vi "Beep.vi"(7 "Enable":bool=TRUE, 8 "Error In":errorcluster, 9 "Beep duration\n(sec)":dbl=0.15, 11 "Beep * n?":i32=1) -> (0 "Error Out":errorcluster)   [LabVIEW 2019]
uses:
  <vilib>/Platform/TimedLoop/XDataNode/timing_clust.ctl
  <vilib>/Platform/TimedLoop/XDataNode/nitl_modes.ctl
  <vilib>/Platform/TimedLoop/XDataNode/wakeup.ctl
  <vilib>/platform/TimedLoop/XDataNode/XDataNode.xnode
  WSCbot_V3_Toolkit.lvlibp
  <vilib>/Platform/TimedLoop/XDataNode/XDNodeRunTimeDep.lvlib
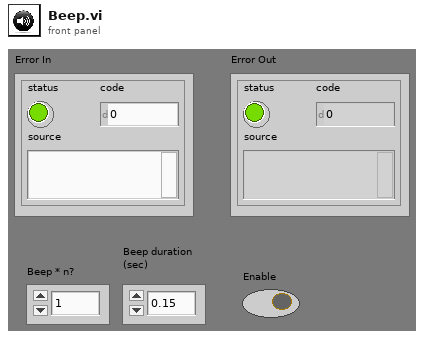
[diagram p1: front panel]
types:
  T1 = typedef "XDNodeRunTimeDep.lvlib/timing_clust.ctl" = cluster{"Expected End [f-1]":u64, "Actual End [f-1]":u64, "Finished Late? [f-1]":bool, "Expected End [i-1]":u64, "Actual End [i-1]":u64, "Finished Late? [i-1]":bool, "Expected Start [i]":u64, "Actual Start [i]":u64, "Expected Start [f]":u64, "Actual Start [f]":u64, "Source Name":string, "Structure Name":string, "Period":i64, "Deadline":i64, "Offset":i64, "Start":i64, "Priority":i32, "Timeout":i32, "Mode":T2, "Wakeup Reason":T3, "Error":errorcluster, "Source Type":string, "Secondary Source Type":string, "Global End Time":u64, "Global Start Time":u64, "Frame Duration":u64, "Iteration Duration":u64, "Assigned CPU":i32, "I/O Scan Engine Mode":u32}
  T2 = typedef "XDNodeRunTimeDep.lvlib/nitl_modes.ctl" = enum32{"No Change", "Process missed periods, maintain original phase", "Discard missed periods, maintain original phase", "Process missed periods, ignore original phase", "Discard missed periods, ignore original phase"}
  T3 = typedef "XDNodeRunTimeDep.lvlib/wakeup.ctl" = enum32{"Normal", "Aborted", "Asynchronous wakeup", "Timing source error", "Timed loop error", "Timeout"}
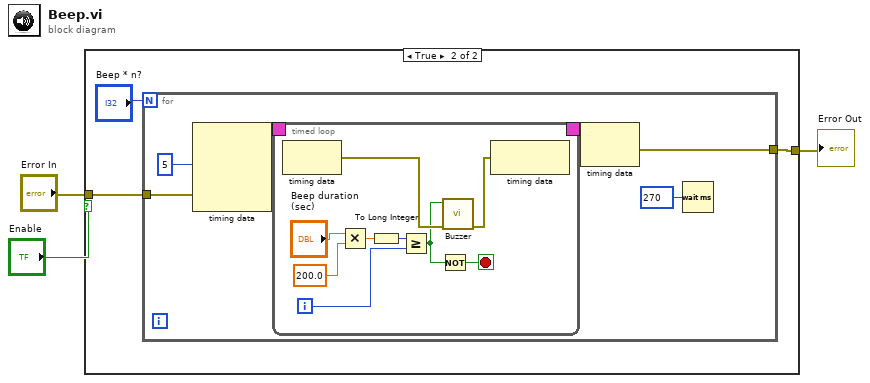
[diagram p0: block diagram]
diagram:
  n1 = case shown="True" "Enable" {
    tunnel: "Error In" -> [w4 w7]
    tunnel: [w4 w6] -> w2
    frame False {
    }
    frame True {
      n2 = for {
        N: "Beep * n?" -> [_]
        tunnel: w7 -> [w11]
        tunnel: [w10] -> w6
        n3 = node-c288(i64 5 ("Period"), w11) -> (w13:T1)  [unwired: 2 in]
        n4 = timed-loop {
          timing: w13 -> [_]
          timing-out: [_] -> w12
          i -> [w20]
          stop <- w19 stop-if-true
          n5 = node-c288() -> (w22:errorcluster)  [unwired: 1 in]
          n6 = Multiply(x="Beep duration\n(sec)", y=200.0 ("x")) -> (x*y=w15:dbl)
          n7 = To Long Integer(number=w15) -> (32bit integer=w14:i32)
          n8 = Greater Or Equal?(x=w14, y=w20) -> (x >= y?=w18:bool)
          n9 = Not(x=w18) -> (.not. x?=w19:bool)
          n10 = call "Buzzer.vi"("error in"=w22, "Set"=w18) -> ("error out"=w21:errorcluster)  [unwired: 9 in]
          n11 = node-c288(w21) -> ()  [unwired: 1 out]
        }
        n12 = node-c288(w12) -> (w10:errorcluster)
        n13 = Wait (ms)(milliseconds to wait=u32 270) -> ()  [unwired: 1 out]
      }
    }
  }
  "Error Out" <- w2
